vi "Get Elo Rating.vi"(11 "Name":string) -> (3 "Rating":i32)   [LabVIEW 2014]
uses:
  <vilib>/Utility/file.llb/Read From Spreadsheet File (string).vi
panel:
  out "size(s)":i32[](array[numeric])
  in  "Path":path=path "C:/Users/Justin/Desktop/LabVIEW-Rank/LabView Contests/Results/Elo_Ratings.csv"
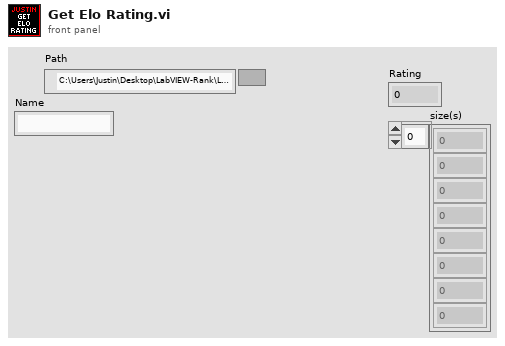
[diagram p1: front panel]
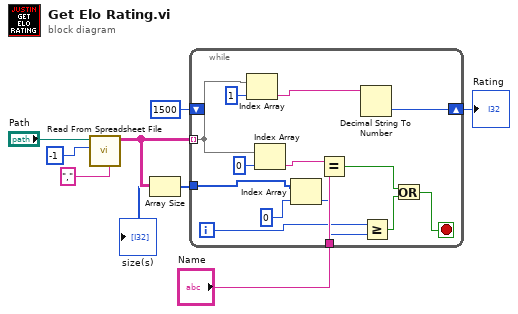
[diagram p0: block diagram]
diagram:
  n1 = call-poly <vilib>:"Read From Spreadsheet File.vi"("delimiter (\\t)"="," ("delimiter (\\t)"), "number of rows (all:-1)"=-1, "file path (dialog if empty)"="Path") -> ("all rows"=w4:string[][])  [unwired: 4 in, 4 out]
  n2 = Array Size(array=w4) -> (size(s)=w3:i32[])
  "size(s)" <- w3
  n3 = while {
    tunnel: w4 -> [w20] mode=indexing
    tunnel: "Name" -> [w16]
    tunnel: w3 -> [w10]
    shift-right: [w18] -> w1
    shift-left: 1500 -> [_]
    i -> [w12]
    stop <- w13 stop-if-true
    n4 = Index Array(array=w20, index=1) -> (element=w19:string)
    n5 = Index Array(array=w20, index=0) -> (element=w17:string)
    n6 = Index Array(array=w10, index=0) -> (element=w9:i32)
    n7 = Equal?(x=w17, y=w16) -> (x = y?=w15:bool)
    n8 = Decimal String To Number(string=w19) -> (number=w18:i32)  [unwired: 2 in, 1 out]
    n9 = Greater Or Equal?(x=w12, y=w9) -> (x >= y?=w14:bool)
    n10 = Or(x=w15, y=w14) -> (x .or. y?=w13:bool)
  }
  "Rating" <- w1
